vi "LCOS Images Init.vi"(2 "LCOS Pattern Display.vi Name":string="LCOS Pattern Display_red.vi", 3 "error in (no error)":errorcluster) -> (6 "Images":T1, 9 "error out":errorcluster)   [LabVIEW 2011]
uses:
  LCOS Images.ctl
  <vilib>/vision/Image Controls.llb/IMAQ Image.ctl
  <vilib>/vision/NI_Vision_Development_Module.lvlib
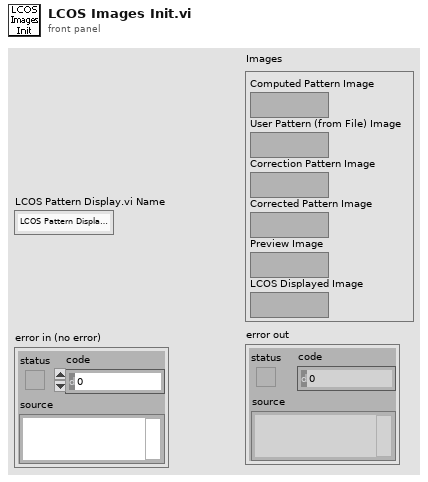
[diagram p1: front panel]
types:
  T1 = typedef "LCOS Images.ctl" = cluster{"Computed Pattern Image":T2, "User Pattern (from File) Image":T2, "Correction Pattern Image":T2, "Corrected Pattern Image":T2, "Preview Image":T2, "LCOS Displayed Image":T2}
  T2 = typedef "IMAQ Image.ctl" = refnum<image>
  T3 = typedef "Image Type" = u32
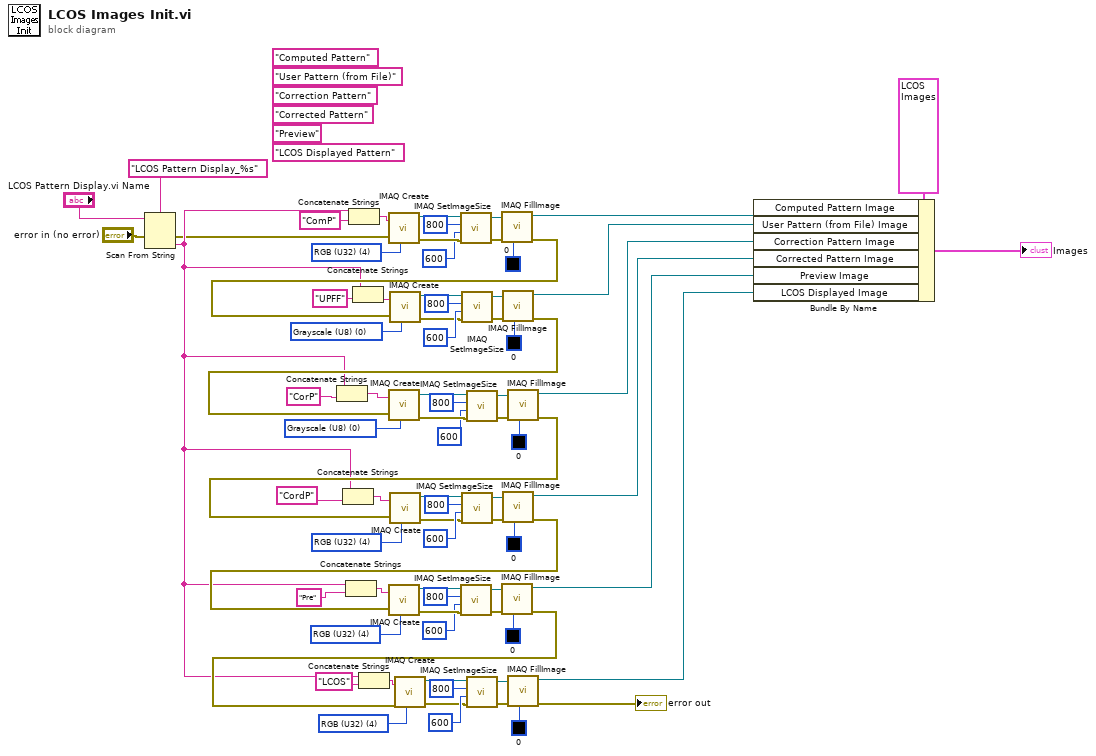
[diagram p0: block diagram]
diagram:
  (unwired) "LCOS Displayed Pattern" ("Image Name")
  (unwired) "Preview" ("Image Name")
  (unwired) "Corrected Pattern" ("Image Name")
  (unwired) "Correction Pattern" ("Image Name")
  (unwired) "User Pattern (from File)" ("Image Name")
  (unwired) "Computed Pattern" ("Image Name")
  w15 = T3 4 items=["Grayscale (U8)", "Grayscale (I16)", "Grayscale (SGL)", "Complex (CSG)", "RGB (U32)", "HSL (U32)", "RGB (U64)", "Grayscale (U16)"] ("Image Type")
  w43 = T3 4 items=["Grayscale (U8)", "Grayscale (I16)", "Grayscale (SGL)", "Complex (CSG)", "RGB (U32)", "HSL (U32)", "RGB (U64)", "Grayscale (U16)"] ("Image Type")
  w44 = T3 4 items=["Grayscale (U8)", "Grayscale (I16)", "Grayscale (SGL)", "Complex (CSG)", "RGB (U32)", "HSL (U32)", "RGB (U64)", "Grayscale (U16)"] ("Image Type")
  w52 = T3 0 items=["Grayscale (U8)", "Grayscale (I16)", "Grayscale (SGL)", "Complex (CSG)", "RGB (U32)", "HSL (U32)", "RGB (U64)", "Grayscale (U16)"] ("Image Type")
  w72 = T3 0 items=["Grayscale (U8)", "Grayscale (I16)", "Grayscale (SGL)", "Complex (CSG)", "RGB (U32)", "HSL (U32)", "RGB (U64)", "Grayscale (U16)"] ("Image Type")
  w63 = T3 4 items=["Grayscale (U8)", "Grayscale (I16)", "Grayscale (SGL)", "Complex (CSG)", "RGB (U32)", "HSL (U32)", "RGB (U64)", "Grayscale (U16)"] ("Image Type")
  n1 = Scan From String(format string="LCOS Pattern Display_%s" ("search string/char (-)"), input string="LCOS Pattern Display.vi Name", error in="error in (no error)") -> (error out=w1:errorcluster, output 1=w3:string)  [unwired: 2 in, 2 out]
  n2 = Concatenate Strings(w3, "CorP" ("Image Name")) -> (w9:string)
  n3 = Concatenate Strings(w3, "CordP" ("Image Name")) -> (w8:string)
  n4 = Concatenate Strings(w3, "Pre" ("Image Name")) -> (w7:string)
  n5 = Concatenate Strings(w3, "ComP" ("Image Name")) -> (w11:string)
  n6 = Concatenate Strings(w3, "UPFF" ("Image Name")) -> (w10:string)
  n7 = Concatenate Strings(w3, "LCOS" ("Image Name")) -> (w6:string)
  n8 = call "IMAQ Create"("Image Name"=w11, "Image Type"=w63, "error in (no error)"=w1) -> ("New Image"=w64:T2, "error out"=w67:errorcluster)  [unwired: 2 in]
  n9 = call "IMAQ SetImageSize"("error in (no error)"=w67, "Y Resolution"=600, "X Resolution"=800, "Image"=w64) -> ("error out"=w69:errorcluster, "Image Out"=w68:T2)  [unwired: 1 in]
  n10 = call "IMAQ FillImage"("Color Pixel Value"=u32 0, "error in (no error)"=w69, "Image"=w68) -> ("error out"=w34:errorcluster, "Image Out"=w29:T2)  [unwired: 7 in]
  n11 = call "IMAQ Create"("Image Name"=w10, "Image Type"=w52, "error in (no error)"=w34) -> ("New Image"=w51:T2, "error out"=w48:errorcluster)  [unwired: 2 in]
  n12 = call "IMAQ SetImageSize"("error in (no error)"=w48, "Y Resolution"=600, "X Resolution"=800, "Image"=w51) -> ("error out"=w46:errorcluster, "Image Out"=w47:T2)  [unwired: 1 in]
  n13 = call "IMAQ FillImage"("Color Pixel Value"=u32 0, "error in (no error)"=w46, "Image"=w47) -> ("error out"=w33:errorcluster, "Image Out"=w28:T2)  [unwired: 7 in]
  n14 = call "IMAQ Create"("Image Name"=w9, "Image Type"=w72, "error in (no error)"=w33) -> ("New Image"=w78:T2, "error out"=w79:errorcluster)  [unwired: 2 in]
  n15 = call "IMAQ SetImageSize"("error in (no error)"=w79, "Y Resolution"=600, "X Resolution"=800, "Image"=w78) -> ("error out"=w74:errorcluster, "Image Out"=w75:T2)  [unwired: 1 in]
  n16 = call "IMAQ FillImage"("Color Pixel Value"=u32 0, "error in (no error)"=w74, "Image"=w75) -> ("error out"=w13:errorcluster, "Image Out"=w27:T2)  [unwired: 7 in]
  n17 = call "IMAQ Create"("Image Name"=w8, "Image Type"=w15, "error in (no error)"=w13) -> ("New Image"=w23:T2, "error out"=w20:errorcluster)  [unwired: 2 in]
  n18 = call "IMAQ SetImageSize"("error in (no error)"=w20, "Y Resolution"=600, "X Resolution"=800, "Image"=w23) -> ("error out"=w18:errorcluster, "Image Out"=w19:T2)  [unwired: 1 in]
  n19 = call "IMAQ FillImage"("Color Pixel Value"=u32 0, "error in (no error)"=w18, "Image"=w19) -> ("error out"=w14:errorcluster, "Image Out"=w12:T2)  [unwired: 7 in]
  n20 = call "IMAQ Create"("Image Name"=w7, "Image Type"=w43, "error in (no error)"=w14) -> ("New Image"=w35:T2, "error out"=w38:errorcluster)  [unwired: 2 in]
  n21 = call "IMAQ SetImageSize"("error in (no error)"=w38, "Y Resolution"=600, "X Resolution"=800, "Image"=w35) -> ("error out"=w40:errorcluster, "Image Out"=w39:T2)  [unwired: 1 in]
  n22 = call "IMAQ FillImage"("Color Pixel Value"=u32 0, "error in (no error)"=w40, "Image"=w39) -> ("error out"=w32:errorcluster, "Image Out"=w26:T2)  [unwired: 7 in]
  n23 = call "IMAQ Create"("Image Name"=w6, "Image Type"=w44, "error in (no error)"=w32) -> ("New Image"=w61:T2, "error out"=w58:errorcluster)  [unwired: 2 in]
  n24 = call "IMAQ SetImageSize"("error in (no error)"=w58, "Y Resolution"=600, "X Resolution"=800, "Image"=w61) -> ("error out"=w56:errorcluster, "Image Out"=w57:T2)  [unwired: 1 in]
  n25 = call "IMAQ FillImage"("Color Pixel Value"=u32 0, "error in (no error)"=w56, "Image"=w57) -> ("error out"=→"error out":errorcluster, "Image Out"=w25:T2)  [unwired: 7 in]
  n26 = Bundle By Name(cluster=T1 {"Computed Pattern Image"=refnum, "User Pattern (from File) Image"=refnum, "Correction Pattern Image"=refnum, "Corrected Pattern Image"=refnum, "Preview Image"=refnum, "LCOS Displayed Image"=refnum} ("Images"), "Computed Pattern Image"=w29, "User Pattern (from File) Image"=w28, "Correction Pattern Image"=w27, "Corrected Pattern Image"=w12, "Preview Image"=w26, "LCOS Displayed Image"=w25) -> (→"Images":T1)
